vi "multi_port.vi"() -> ()   [LabVIEW 2016]
uses:
  dxl_x86_c.lvlib/dxl_x86_c.lvlib
panel:
  out "dynamixel2_error":string
  out "dynamixel2_comm_result":string
  out "dynamixel1_error":string
  out "dynamixel1_comm_result":string
  out "value : PRO (knob)\npresent position 2":i32(knob) scale=150000.0..-150000.0
  in  "device_name2":string="COM2"
  out "port_num2":i32=1
  in  "dynamixe2_id":u8=2
  in  "device_name1":string="COM1"
  in  "ADDR_PRO_\nPRESENT_POSITION":u16=611
  in  "ADDR_PRO_\nGOAL_POSITION":u16=596
  in  "ADDR_PRO_\nTORQUE_ENABLE":u16=562
  out "protocol_version":dbl=2.0
  out "value : PRO (knob)\npresent position 1":i32(knob) scale=150000.0..-150000.0
  in  "terminate":bool
  out "port_num1":i32
  in  "value : PRO (dial)\ngoal position":i32(knob) scale=150000.0..-150000.0
  in  "dynamixel1_id":u8=1
  in  "baud_rate":i32=57600
  # "/*******************************************************************************\n* Copyright (c) 2016, ROBOTIS CO., LTD.\n* All rights reserved.\n*\n* Redistribution and use in source and binary forms, with or without\n* modification, are permitted provided that the following conditions are met:\n*\n* * Redistributions of source code must retain the above copyright notice, this\n*   list of conditions and the following disclaimer.\n*\n* * Redistributions in binary form must reproduce the above copyright notice,\n*   this list of conditions and the following disclaimer in the documentation\n*   and/or other materials provided with the distribution.\n*\n* * Neither the name of ROBOTIS nor the names of its\n*   contributors may be used to endorse or promote products derived from\n*   this software without specific prior written permission.\n*\n* THIS SOFTWARE IS PROVIDED BY THE COPYRIGHT HOLDERS AND CONTRIBUTORS \"AS IS\"\n* AND ANY EXPRESS OR IMPLIED WARRANTIES, INCLUDING, BUT NOT LIMITED TO, THE\n* IMPLIED WARRANTIES OF MERCHANTABILITY AND FITNESS FOR A PARTICULAR PURPOSE ARE\n* DISCLAIMED. IN NO EVENT SHALL THE COPYRIGHT HOLDER OR CONTRIBUTORS BE LIABLE\n* FOR ANY DIRECT, INDIRECT, INCIDENTAL, SPECIAL, EXEMPLARY, OR CONSEQUENTIAL\n* DAMAGES (INCLUDING, BUT NOT LIMITED TO, PROCUREMENT OF SUBSTITUTE GOODS OR\n* SERVICES; LOSS OF USE, DATA, OR PROFITS; OR BUSINESS INTERRUPTION) HOWEVER\n* CAUSED AND ON ANY THEORY OF LIABILITY, WHETHER IN CONTRACT, STRICT LIABILITY,\n* OR TORT (INCLUDING NEGLIGENCE OR OTHERWISE) ARISING IN ANY WAY OUT OF THE USE\n* OF THIS SOFTWARE, EVEN IF ADVISED OF THE POSSIBILITY OF SUCH DAMAGE.\n*******************************************************************************/\n\n/* Author: Ryu Woon Jung (Leon) */"
  # "Available Dynamixel model on this example : All models using Protocol 2.0\nThis example is designed for using two Dynamixel PRO 54-200, and two USB2DYNAMIXEL.\nTo use another Dynamixel model, such as X series, see their details in E-Manual(support.robotis.com) \n   and edit \"numeric control\"s seen left with \"Edit Text\" tool.\nBe sure that Dynamixel PRO properties are already set as %% ID : 1 / Baudnum : 1 (Baudrate : 57600)\n\n\n1. Run example by click above \"Run\" button (below \"Edit\" menu).\n2. Drag \"dial\" then you may see the Dynamixel and \"knob\"s rotating\n3. To finish the example, press \"terminate\" button."
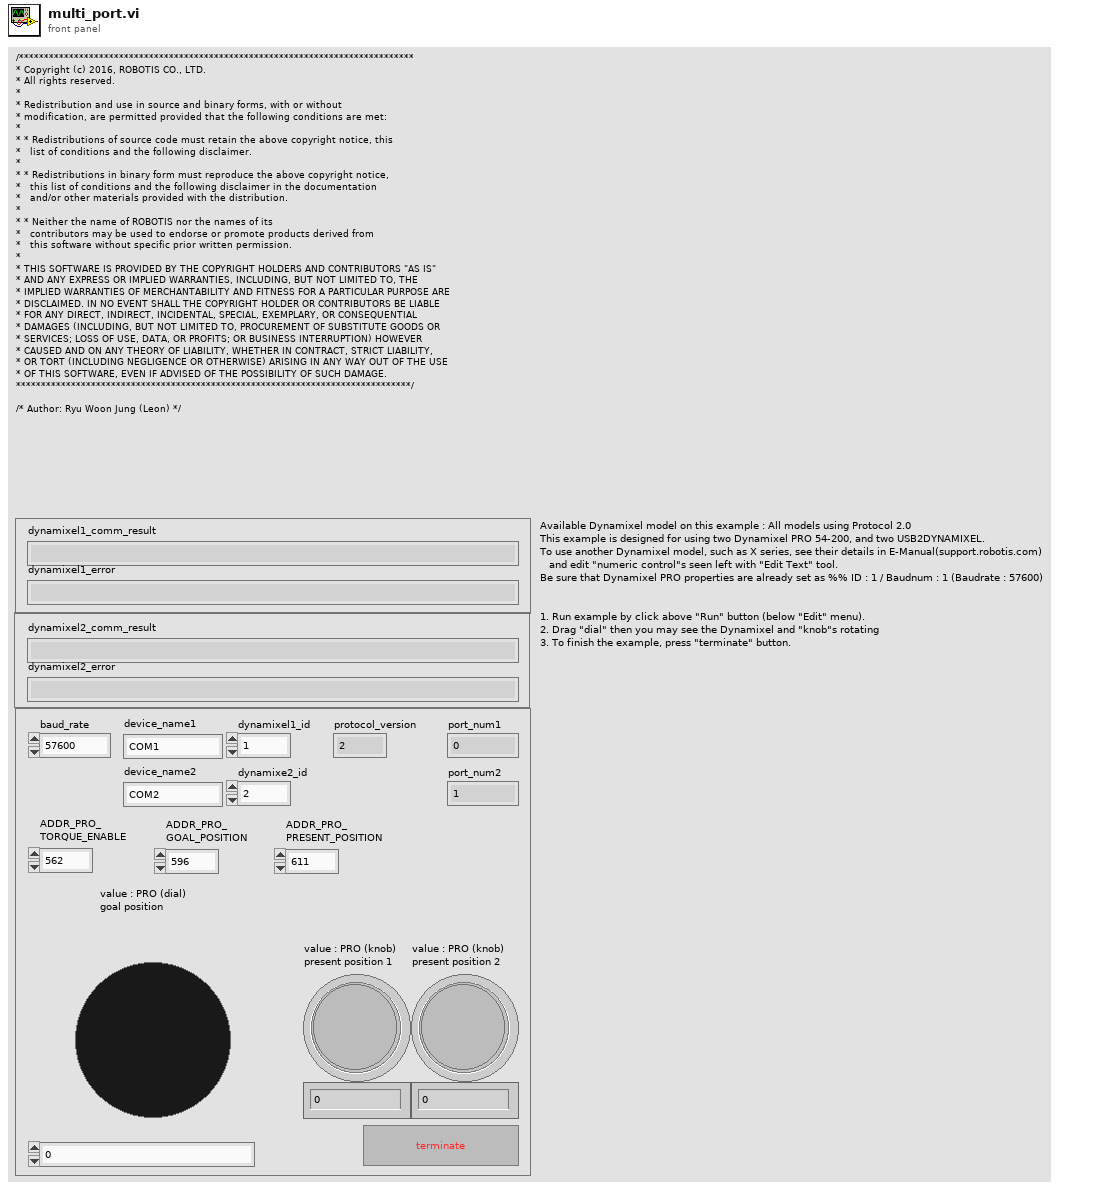
[diagram p1: front panel]
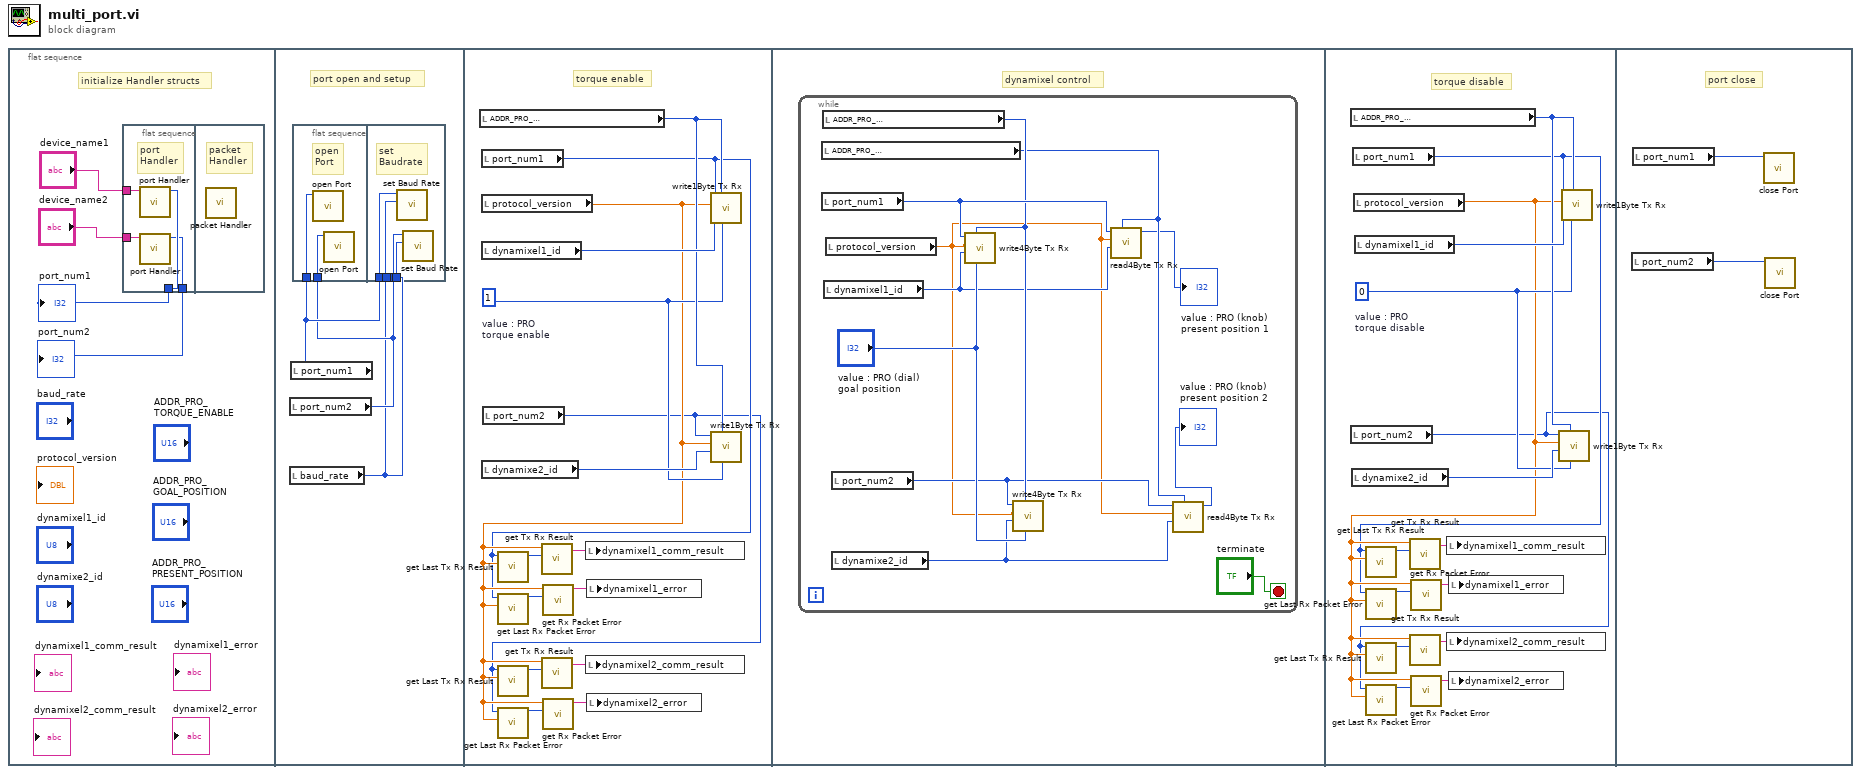
[diagram p0: block diagram]
diagram:
  n1 = flat-sequence {
    frame #0 {
      # "initialize Handler structs"
      n2 = flat-sequence {
        tunnel: "device_name1" -> [w8]
        tunnel: "device_name2" -> [w7]
        tunnel: [w6] -> w2
        tunnel: [w5] -> w1
        frame #0 {
          # "port\nHandler"
          n3 = call "port Handler.vi"("port_name"=w8) -> ("function return"=w6:i32)  [unwired: 10 in]
          n4 = call "port Handler.vi"("port_name"=w7) -> ("function return"=w5:i32)  [unwired: 10 in]
        }
        frame #1 {
          # "packet\nHandler"
          n5 = call "packet Handler.vi"() -> ()  [unwired: 12 in]
        }
      }
      "port_num1" <- w2
      "port_num2" <- w1
    }
    frame #1 {
      # "port open and setup"
      n6 = local read "port_num2"() -> (w10:i32)
      n7 = local read "baud_rate"() -> (w9:i32)
      n8 = local read "port_num1"() -> (w11:i32)
      n9 = flat-sequence {
        tunnel: w11 -> [w13]
        tunnel: w10 -> [w12]
        tunnel: w11 -> [w17]
        tunnel: w9 -> [w16]
        tunnel: w10 -> [w15]
        tunnel: w9 -> [w14]
        frame #0 {
          # "open\nPort"
          n10 = call "open Port.vi"("port_num"=w13) -> ()  [unwired: 10 in, 1 out]
          n11 = call "open Port.vi"("port_num"=w12) -> ()  [unwired: 10 in, 1 out]
        }
        frame #1 {
          # "set\nBaudrate"
          n12 = call "set Baud Rate.vi"("baudrate"=w16, "port_num"=w17) -> ()  [unwired: 9 in, 1 out]
          n13 = call "set Baud Rate.vi"("baudrate"=w14, "port_num"=w15) -> ()  [unwired: 9 in, 1 out]
        }
      }
    }
    frame #2 {
      w29 = 1  # value : PRO torque enable
      # "torque enable"
      n14 = local read "ADDR_PRO_\nTORQUE_ENABLE"() -> (w31:u16)
      n15 = local read "port_num1"() -> (w19:i32)
      n16 = local read "protocol_version"() -> (w20:dbl)
      n17 = local read "dynamixel1_id"() -> (w32:u8)
      n18 = local read "dynamixe2_id"() -> (w30:u8)
      n19 = local read "port_num2"() -> (w18:i32)
      n20 = call "get Last Tx Rx Result.vi"("protocol_version"=w20, "port_num"=w19) -> ("function return"=w25:i32)  [unwired: 9 in]
      n21 = call "get Last Rx Packet Error.vi"("protocol_version"=w20, "port_num"=w19) -> ("function return"=w26:u8)  [unwired: 9 in]
      n22 = call "get Last Tx Rx Result.vi"("protocol_version"=w20, "port_num"=w18) -> ("function return"=w24:i32)  [unwired: 9 in]
      n23 = call "get Last Rx Packet Error.vi"("protocol_version"=w20, "port_num"=w18) -> ("function return"=w23:u8)  [unwired: 9 in]
      n24 = call "get Tx Rx Result.vi"("result"=w25, "protocol_version"=w20) -> ("function return"=w28:string)  [unwired: 9 in]
      n25 = call "get Tx Rx Result.vi"("result"=w24, "protocol_version"=w20) -> ("function return"=w21:string)  [unwired: 9 in]
      n26 = call "get Rx Packet Error.vi"("error"=w26, "protocol_version"=w20) -> ("function return"=w27:string)  [unwired: 9 in]
      n27 = call "get Rx Packet Error.vi"("error"=w23, "protocol_version"=w20) -> ("function return"=w22:string)  [unwired: 9 in]
      n28 = local write "dynamixel1_comm_result"(w28) -> ()
      n29 = local write "dynamixel2_comm_result"(w21) -> ()
      n30 = local write "dynamixel1_error"(w27) -> ()
      n31 = local write "dynamixel2_error"(w22) -> ()
      n32 = call "write1Byte Tx Rx.vi"("data"=w29, "address"=w31, "id"=w32, "protocol_version"=w20, "port_num"=w19) -> ()  [unwired: 7 in]
      n33 = call "write1Byte Tx Rx.vi"("data"=w29, "address"=w31, "id"=w30, "protocol_version"=w20, "port_num"=w18) -> ()  [unwired: 7 in]
    }
    frame #3 {
      # "dynamixel control"
      n34 = while {
        stop <- "terminate" stop-if-true
        n35 = local read "ADDR_PRO_\nPRESENT_POSITION"() -> (w38:u16)
        n36 = local read "port_num1"() -> (w42:i32)
        n37 = local read "ADDR_PRO_\nGOAL_POSITION"() -> (w40:u16)
        n38 = local read "dynamixel1_id"() -> (w39:u8)
        n39 = local read "protocol_version"() -> (w33:dbl)
        n40 = local read "port_num2"() -> (w34:i32)
        n41 = local read "dynamixe2_id"() -> (w35:u8)
        n42 = call "write4Byte Tx Rx.vi"("data"="value : PRO (dial)\ngoal position", "address"=w40, "id"=w39, "protocol_version"=w33, "port_num"=w42) -> ()  [unwired: 7 in]
        n43 = call "write4Byte Tx Rx.vi"("data"="value : PRO (dial)\ngoal position", "address"=w40, "id"=w35, "protocol_version"=w33, "port_num"=w34) -> ()  [unwired: 7 in]
        n44 = call "read4Byte Tx Rx.vi"("address"=w38, "id"=w39, "protocol_version"=w33, "port_num"=w42) -> ("function return"=→"value : PRO (knob)\npresent position 1":u32)  [unwired: 7 in]
        n45 = call "read4Byte Tx Rx.vi"("address"=w38, "id"=w35, "protocol_version"=w33, "port_num"=w34) -> ("function return"=→"value : PRO (knob)\npresent position 2":u32)  [unwired: 7 in]
      }
    }
    frame #4 {
      w55 = 0  # value : PRO torque disable
      # "torque disable"
      n46 = local read "ADDR_PRO_\nTORQUE_ENABLE"() -> (w57:u16)
      n47 = local read "port_num2"() -> (w44:i32)
      n48 = local read "dynamixe2_id"() -> (w56:u8)
      n49 = local read "port_num1"() -> (w45:i32)
      n50 = local read "protocol_version"() -> (w46:dbl)
      n51 = local read "dynamixel1_id"() -> (w58:u8)
      n52 = call "get Last Tx Rx Result.vi"("protocol_version"=w46, "port_num"=w45) -> ("function return"=w52:i32)  [unwired: 9 in]
      n53 = call "get Last Rx Packet Error.vi"("protocol_version"=w46, "port_num"=w45) -> ("function return"=w51:u8)  [unwired: 9 in]
      n54 = call "get Last Tx Rx Result.vi"("protocol_version"=w46, "port_num"=w44) -> ("function return"=w49:i32)  [unwired: 9 in]
      n55 = call "get Last Rx Packet Error.vi"("protocol_version"=w46, "port_num"=w44) -> ("function return"=w50:u8)  [unwired: 9 in]
      n56 = call "get Tx Rx Result.vi"("result"=w52, "protocol_version"=w46) -> ("function return"=w53:string)  [unwired: 9 in]
      n57 = call "get Tx Rx Result.vi"("result"=w49, "protocol_version"=w46) -> ("function return"=w48:string)  [unwired: 9 in]
      n58 = call "get Rx Packet Error.vi"("error"=w51, "protocol_version"=w46) -> ("function return"=w54:string)  [unwired: 9 in]
      n59 = call "get Rx Packet Error.vi"("error"=w50, "protocol_version"=w46) -> ("function return"=w47:string)  [unwired: 9 in]
      n60 = local write "dynamixel1_comm_result"(w53) -> ()
      n61 = local write "dynamixel2_comm_result"(w48) -> ()
      n62 = local write "dynamixel1_error"(w54) -> ()
      n63 = local write "dynamixel2_error"(w47) -> ()
      n64 = call "write1Byte Tx Rx.vi"("data"=w55, "address"=w57, "id"=w56, "protocol_version"=w46, "port_num"=w44) -> ()  [unwired: 7 in]
      n65 = call "write1Byte Tx Rx.vi"("data"=w55, "address"=w57, "id"=w58, "protocol_version"=w46, "port_num"=w45) -> ()  [unwired: 7 in]
    }
    frame #5 {
      # "port close"
      n66 = local read "port_num2"() -> (w59:i32)
      n67 = local read "port_num1"() -> (w60:i32)
      n68 = call "close Port.vi"("port_num"=w60) -> ()  [unwired: 11 in]
      n69 = call "close Port.vi"("port_num"=w59) -> ()  [unwired: 11 in]
    }
  }
